vi "set bindy key.vi"(8 "error in (no error)":errorcluster, 11 "keyfilepath":string) -> (0 "error out":errorcluster, 3 "function return":i32)   [LabVIEW 2012, in "libximc.lvlib"]
doc: "result_t XIMC_API set_bindy_key(const char* keyfilepath);"
uses:
  libximc.lvlib
  libximc.dll
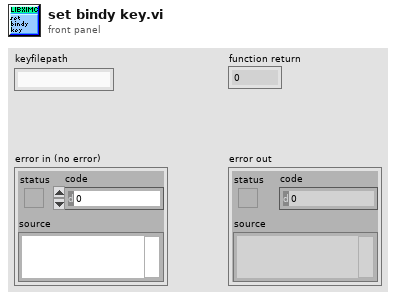
[diagram p1: front panel]
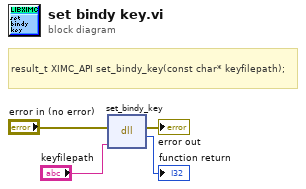
[diagram p0: block diagram]
diagram:
  # "result_t XIMC_API set_bindy_key(const char* keyfilepath);"
  n1 = dll-call lib="C:/Users/user/Desktop/labview-2.9.11-gen/libximc.*" fn="set_bindy_key"(error in="error in (no error)", "keyfilepath"="keyfilepath") -> (error out=→"error out":errorcluster, →"function return":i32)  [unwired: 3 in, 1 out]
